vi "ZDS1104 Config.vi"(9 "参数":T1={"Coupling Mode (1: DC)"=1, "Probe"=9, "datebase"=enum."10ms", "volbase(V)"=5.0} {"Probe" items=["0.001", "0.002", "0.005", "0.01", "0.02", "0.05", "0.1", "0.2", "0.5", "1", "2", "5", "10", "20", "50", "100", "200", "500", "1000"]; "Coupling Mode (1: DC)" items=["AC", "DC", "GND"]}, 10 "Channel":i32(ring)=1 items=["Channel 1"=1, "Channel 2"=2, "Channel 3"=3, "Channel 4"=4], 11 "MyIndex":u8) -> (0 "error out":errorcluster caption="错误输出", 3 "ok?":bool)   [LabVIEW 2015]
uses:
  ZhiYuan ZDS Series for TCP/ZhiYuan ZDS Series for TCP.lvlib
panel:
  in  "错误输入":errorcluster
  out "VISA":refnum<visa-resource-name> caption="VISA资源名称输出"
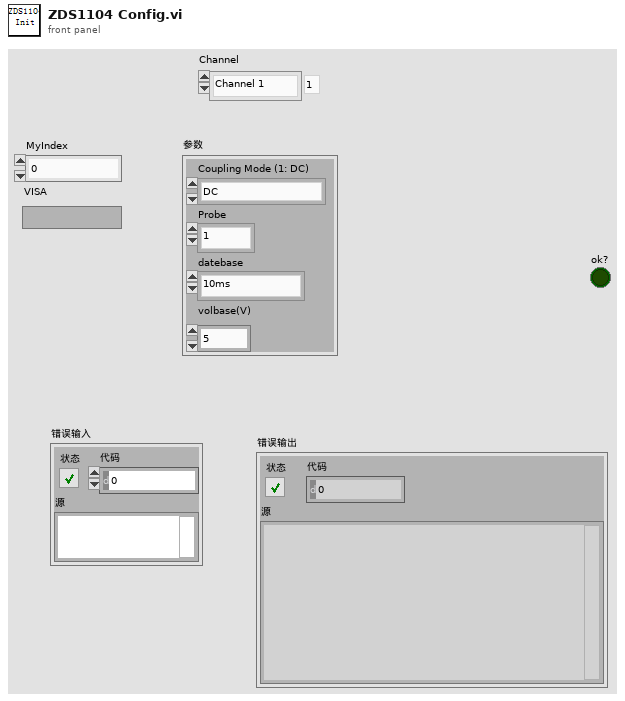
[diagram p1: front panel]
types:
  T1 = cluster{"Coupling Mode (1: DC)":i32, "Probe":i32, "datebase":enum16{"1ns", "2ns", "5ns", "10ns", "20ns", "50ns", "100ns", "200ns", "500ns", "1us", "2us", "5us", "10us", "20us", "50us", "100us", "200us", "500us", "1ms", "2ms", "5ms", "10ms", "20ms", "50ms", "100ms", "200ms", "500ms", "1s", "2s", "5s", "10s", "20s", "50s", "100s"}, "volbase(V)":dbl}
  T2 = enum16{"1ns", "2ns", "5ns", "10ns", "20ns", "50ns", "100ns", "200ns", "500ns", "1us", "2us", "5us", "10us", "20us", "50us", "100us", "200us", "500us", "1ms", "2ms", "5ms", "10ms", "20ms", "50ms", "100ms", "200ms", "500ms", "1s", "2s", "5s", "10s", "20s", "50s", "100s"}
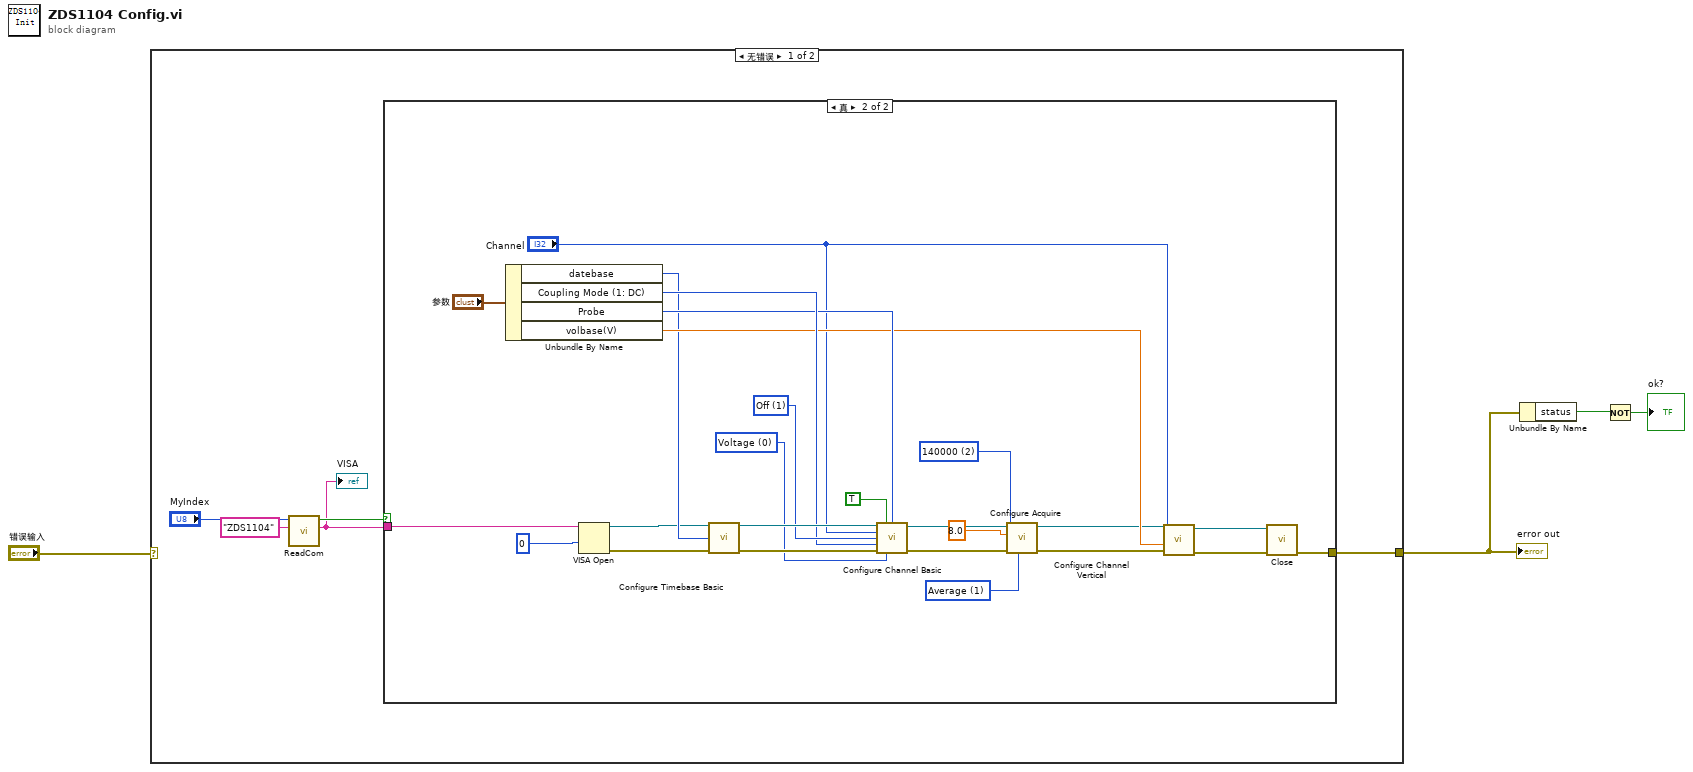
[diagram p0: block diagram]
diagram:
  n1 = case shown="无错误" "错误输入" {
    selector: "错误输入" -> [_ w35]
    tunnel: [w9 w35] -> w2
    frame No Error {
      n2 = call "ReadCom.vi"("仪器名称"="ZDS1104", "MyIndex"="MyIndex") -> ("COM"=w5:string, "OK?"=w6:bool)  [unwired: 7 in, 1 out]
      "VISA" <- w5
      n3 = case shown="真" w6 {
        tunnel: [_ w11] -> w9
        tunnel: w5 -> [_ w13]
        frame False {
        }
        frame True {
          w17 = 2 items=["Auto", "14000", "140000", "1400000", "14000000", "56000000", "112000000", "3500", "7000", "70000", "700000", "7000000", "28000000"] ("Waveform Point Number (0: Auto)")
          w18 = 1 items=["Normal", "Average", "Peak", "High Resolution"] ("Acquisition Mode (0: Normal)")
          w30 = 0 items=["Voltage", "Ampere"] ("Unit (0: Voltage)")
          w31 = 1 items=["20M", "Off"] ("Bandwidth Limit")
          n4 = Unbundle By Name("参数") -> ("datebase"=w23:T2, "Coupling Mode (1: DC)"=w27:i32, "Probe"=w26:i32, "volbase(V)"=w25:dbl)
          n5 = VISA Open(access mode=u32 0, VISA resource name=w13) -> (VISA resource name=w15:refnum<visa-resource-name>, error out=w14:errorcluster)  [unwired: 3 in]
          n6 = call "Configure Timebase Basic.vi"("VISA resource name"=w15, "Scale"=w23, "error in (no error)"=w14) -> ("VISA resource name out"=w33:refnum<visa-resource-name>, "error out"=w34:errorcluster)  [unwired: 11 in]
          n7 = call "Configure Channel Basic.vi"("VISA resource name"=w33, "Enable Channel (F: Disable)"=TRUE, "Probe"=w26, "Channel (1: Channel 1)"="Channel", "Bandwidth Limit"=w31, "Coupling Mode (1: DC)"=w27, "error in (no error)"=w34, "Unit (0: Voltage)"=w30) -> ("VISA resource name out"=w21:refnum<visa-resource-name>, "error out"=w29:errorcluster)  [unwired: 6 in]
          n8 = call "Configure Acquire.vi"("Acquisition Mode (0: Normal)"=w18, "error in (no error)"=w29, "Waveform Point Number (0: Auto)"=w17, "Average Number (2)"=8.0, "VISA resource name"=w21) -> ("error out"=w22:errorcluster, "VISA resource name out"=w20:refnum<visa-resource-name>)  [unwired: 5 in]
          n9 = call "Configure Channel Vertical.vi"("error in (no error)"=w22, "Scale (1)"=w25, "Channel (1: Channel 1)"="Channel", "VISA resource name"=w20) -> ("error out"=w12:errorcluster, "VISA resource name out"=w10:refnum<visa-resource-name>)  [unwired: 6 in]
          n10 = call "Close.vi"("error in (no error)"=w12, "VISA resource name"=w10) -> ("error out"=w11:errorcluster)  [unwired: 9 in]
        }
      }
    }
    frame Error {
    }
  }
  "error out" <- w2
  n11 = Unbundle By Name(w2) -> ("status"=w4:bool)
  n12 = Not(x=w4) -> (.not. x?=→"ok?":bool)
